vi "Engine In - Specifications.vi"() -> (0 "Q.LHV Fuel [kJ/kg]":sgl, 1 "StoichAFR":sgl, 2 "Engine Displacement (cc)":sgl, 3 "Number of Cylinders":u8)   [LabVIEW 2015, in "ECS-RT.lvlib"]
uses:
  ECS-RT.lvlib
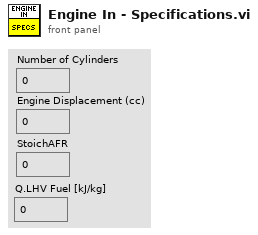
[diagram p1: front panel]
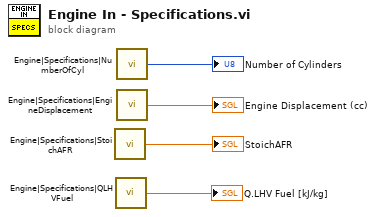
[diagram p0: block diagram]
diagram:
  n1 = call "Engine|Specifications|StoichAFR"() -> ("Value"=→"StoichAFR":sgl)
  n2 = call "Engine|Specifications|QLHVFuel"() -> ("Value"=→"Q.LHV Fuel [kJ/kg]":sgl)
  n3 = call "Engine|Specifications|NumberOfCyl"() -> ("Value"=→"Number of Cylinders":u8)
  n4 = call "Engine|Specifications|EngineDisplacement"() -> ("Value"=→"Engine Displacement (cc)":sgl)
